vi "Logger.Variant.WriteWithBackup.vi"(8 "error in":errorcluster, 9 "header":string, 10 "addition":string, 11 "file":path) -> (0 "error out":errorcluster)   [LabVIEW 2016]
doc: "Writes to a file.\nIf <B>append</B> is false (default), the file will be rewritten.\nIf <B>append</B> is true, the new data will be appended to the file.\nSupports a <B>header</B> line which will be placed on top of the file when it is created or rewritten. This <B>header</B> line requires a newline at the end."
panel:
  # "Added at begin only if file is created"
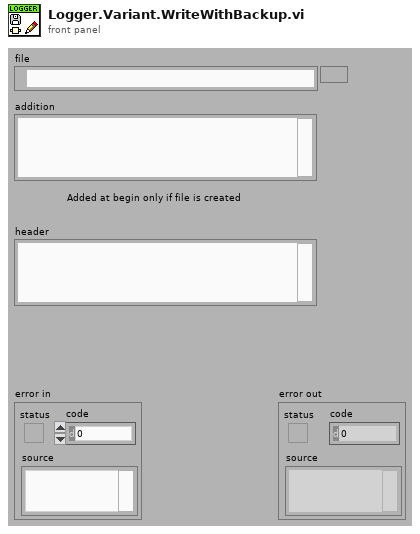
[diagram p1: front panel]
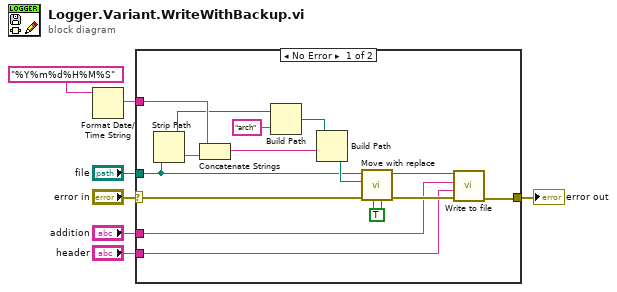
[diagram p0: block diagram]
diagram:
  n1 = Format Date/Time String(time format string (%c)="%Y%m%d%H%M%S") -> (date/time string=w3:string)  [unwired: 2 in]
  n2 = case shown="No Error" "error in" {
    selector: "error in" -> [w15 w22]
    tunnel: [w13 w22] -> w7
    tunnel: "file" -> [w11 _]
    tunnel: "addition" -> [w10 _]
    tunnel: w3 -> [w21 _]
    tunnel: "header" -> [w8 _]
    frame No Error {
      w9 = TRUE ("replace allowed (T)")
      n3 = Strip Path(path=w11) -> (stripped path=w18:path, name=w20:string)
      n4 = Concatenate Strings(w21, w20) -> (w19:string)
      n5 = Build Path(base path=w18, name or relative path="arch") -> (appended path=w16:path)
      n6 = Build Path(base path=w16, name or relative path=w19) -> (appended path=w12:path)
      n7 = call "Move with replace.vi"("create parent dirs (F)"=w9, "replace allowed (T)"=w9, "error in (no error)"=w15, "destination path"=w12, "source path"=w11) -> ("error"=w14:errorcluster)  [unwired: 6 in]
      n8 = call "Write to file.vi"("error in"=w14, "header"=w8, "addition"=w10, "file"=w11) -> ("error out"=w13:errorcluster)  [unwired: 7 in]
    }
    frame Error {
    }
  }
  "error out" <- w7
